vi "Get Parameter Value - Double Float.vi"(7 "Default value":dbl format="%#_13g", 8 "error in (no error)":errorcluster, 9 "Parameter name":string, 10 "Config name":string, 11 "Config in":refnum<class "Config.lvclass">) -> (0 "error out":errorcluster, 2 "Value":dbl, 3 "Config out":refnum<class "Config.lvclass">)   [LabVIEW 2020, in "TALOS.lvlib" / "Classes.lvlib" / "Config.lvclass"]
doc: "Get the parameter's value (double) from the specified configuration"
uses:
  Config.lvclass
  Config.lvclass/Config.ctl
  Ancestor/Ancestor/Ancestor.lvclass/Ancestor.ctl
  FGV/Error Memory/Get Error Description.vi
  Support VIs/Get PC name.vi
  Ancestor/Ancestor/Read ID.vi
  Support VIs/Get Class Name.vi
  <vilib>/Utility/error.llb/Clear Errors.vi
  FGV/Error Memory/Error Memory Core.vi
  <vilib>/AdvancedString/Delimited String to 1D String Array.vi
  Support VIs/Circus Root Path.vi
  FGV/Error Memory/Error Crt Lvl checker.vi
  FGV/Error Memory/Error Memory Core.vi/40c8088d-b597-4017-91af-faa98e00292e.vi
  FGV/Error Memory/Error Memory Core.vi/d4a3ab98-063c-4e44-b43d-fbdcfe6c2be2.vi
  Support VIs/Global Memory.vi
  <vilib>/Utility/LVClass/Get LV Class Name.vi
  Support VIs/Is in Packed Library.vi
  Support VIs/TALOS Root path.vi
  Support VIs/Read CSV worksheet.vi
  Support VIs/Global Constants.vi
  <vilib>/Utility/error.llb/General Error Handler.vi
  Support VIs/Error Log.vi
  Ancestor/Ancestor/Ancestor.lvclass
  <vilib>/Comparison/Equal/Equal Functor/Equal Functor.lvclass
  TALOS.lvlib
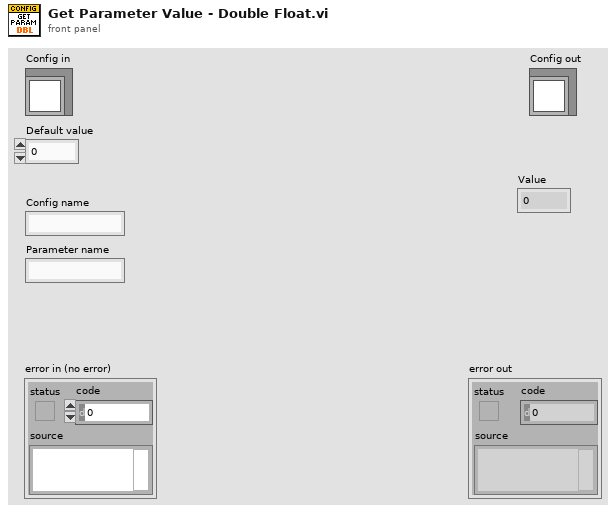
[diagram p1: front panel]
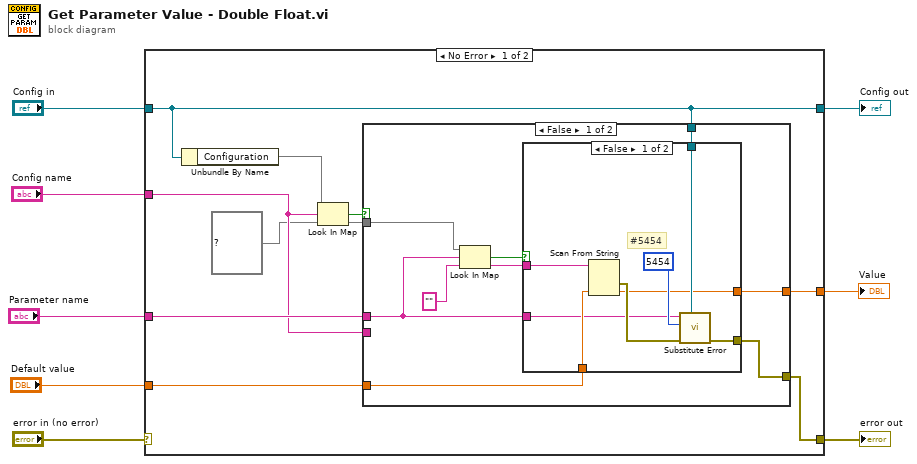
[diagram p0: block diagram]
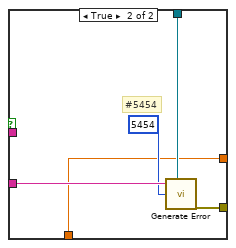
[diagram p2: hidden frame]
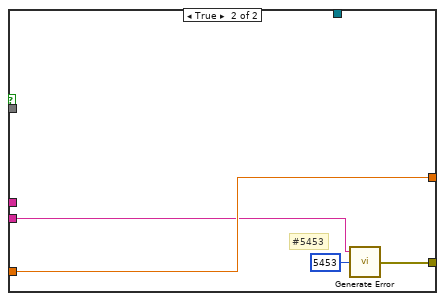
[diagram p3: hidden frame]
diagram:
  n1 = case shown="No Error" "error in (no error)" {
    selector: "error in (no error)" -> [_ w47]
    tunnel: [w15 w47] -> w3
    tunnel: [w12 w46] -> w1
    tunnel: "Config in" -> [w12 w46]
    tunnel: "Parameter name" -> [w16 _]
    tunnel: [w13 w45] -> w2
    tunnel: "Default value" -> [w11 w45]
    tunnel: "Config name" -> [w10 _]
    frame No Error {
      n2 = Unbundle By Name(w12) -> ("Configuration"=w18:map{string, map{string, string}})
      n3 = Look In Map(map=w18, key=w10, default value=map{string, string} {}) -> (key not found?=w14:bool, value=w17:map{string, string})
      n4 = case shown="False" w14 {
        tunnel: w10 -> [_ w41]
        tunnel: w17 -> [w23 _]
        tunnel: w16 -> [w22 _]
        tunnel: [w25 w43] -> w15
        tunnel: [w27 w42] -> w13
        tunnel: w12 -> [w26 _]
        tunnel: w11 -> [w24 w42]
        frame False {
          n5 = Look In Map(map=w23, key=w22, default value="") -> (key not found?=w20:bool, value=w19:string)
          n6 = case shown="False" w20 {
            tunnel: w19 -> [w28 _]
            tunnel: [w30 w36] -> w27
            tunnel: w26 -> [w34 w39]
            tunnel: [w33 w40] -> w25
            tunnel: w22 -> [w29 w38]
            tunnel: w24 -> [w31 w36]
            frame False {
              # "#5454"
              n7 = Scan From String(input string=w28, default 1=w31) -> (error out=w35:errorcluster, output 1=w30:dbl)  [unwired: 3 in, 2 out]
              n8 = call "Substitute Error.vi"("LabVIEW Object"=w34, "error in (no error)"=w35, "Error Code"=5454, "Optional String"=w29) -> ("error out"=w33:errorcluster)  [unwired: 7 in]
            }
            frame True {
              # "#5454"
              n9 = call "Generate Error.vi"("Optional String"=w38, "Class"=w39, "Error Code"=5454) -> ("error out"=w40:errorcluster)  [unwired: 4 in]
            }
          }
        }
        frame True {
          # "#5453"
          n10 = call "Generate Error.vi"("Optional String"=w41, "Error Code"=5453) -> ("error out"=w43:errorcluster)  [unwired: 5 in]
        }
      }
    }
    frame Error {
    }
  }
  "error out" <- w3
  "Config out" <- w1
  "Value" <- w2
